vi "File - Create Directory Path.vi"(8 "error in (no error)":errorcluster, 11 "Path":path) -> (0 "error out":errorcluster, 3 "Path Out":path)   [LabVIEW 2018]
doc: "Creates an entire directory path of any length. All subdirectories in the path are created.\n\nReturns an error if the path cannot be created or does not exist."
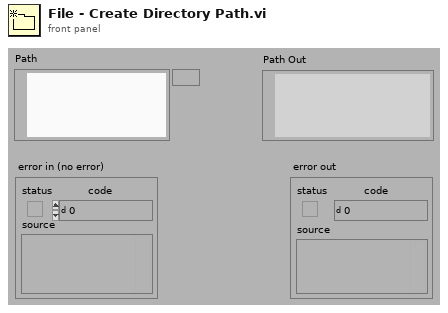
[diagram p1: front panel]
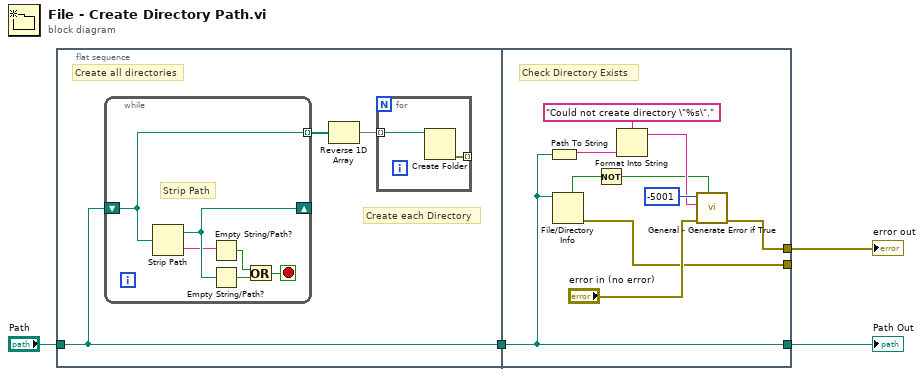
[diagram p0: block diagram]
diagram:
  n1 = flat-sequence {
    tunnel: "Path" -> [w5]
    tunnel: [w5] -> w3
    tunnel: w3 -> [w21]
    tunnel: [w21] -> w2
    tunnel: [w18] -> w1
    tunnel: [w16] -> _
    frame #0 {
      # "Create each Directory"
      # "Create all directories"
      n2 = while {
        tunnel: [w13] -> w7 mode=indexing
        shift-right: [w15] -> _
        shift-left: w5 -> [w13]
        stop <- w12 stop-if-true
        # "Strip Path"
        n3 = Strip Path(path=w13) -> (stripped path=w15:path, name=w10:string)
        n4 = Empty String/Path?(string/path=w10) -> (empty?=w11:bool)
        n5 = Empty String/Path?(string/path=w15) -> (empty?=w14:bool)
        n6 = Or(x=w11, y=w14) -> (x .or. y?=w12:bool)
      }
      n7 = Reverse 1D Array(array=w7) -> (reversed array=w6:path[])
      n8 = for {
        tunnel: w6 -> [w9] mode=indexing
        tunnel: [w8] -> _ mode=indexing
        n9 = Create Folder(path (use dialog)=w9) -> (error out=w8:errorcluster)  [unwired: 2 in, 2 out]
      }
    }
    frame #1 {
      # "Check Directory Exists"
      n10 = Path To String(path=w21) -> (string=w22:string)
      n11 = File/Directory Info(path=w21) -> (directory=w25:bool, error out=w16:errorcluster)  [unwired: 1 in, 5 out]
      n12 = Not(x=w25) -> (.not. x?=w17:bool)
      n13 = Format Into String(format string="Could not create directory \"%s\"." ("String"), w22) -> (resulting string=w23:string)  [unwired: 2 in, 1 out]
      n14 = call "General - Generate Error if True.vi"("Generate Error"=w17, "error in (no error)"="error in (no error)", "String"=w23, "Error (-1000)"=-5001) -> ("error out"=w18:errorcluster)  [unwired: 5 in]
    }
  }
  "Path Out" <- w2
  "error out" <- w1
